vi "DeactivateChnl HW.vi"(8 "error in (no error)":errorcluster, 10 "Chnl Name":string, 11 "BME_DG_G08 in":refnum<class "BME_DG_G08.lvclass">) -> (0 "error out":errorcluster, 3 "BME_DG_G08 out":refnum<class "BME_DG_G08.lvclass">)   [LabVIEW 2009, in "POLARIS BME DG.lvlib" / "BME_DG_G08.lvclass"]
uses:
  BME_DG_G08.lvclass
  BME_DG_G05P2/BME_DG_G05P2.lvclass
  POLARIS BME DG.lvlib
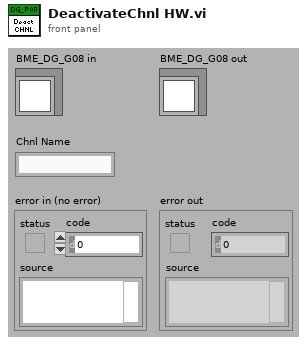
[diagram p1: front panel]
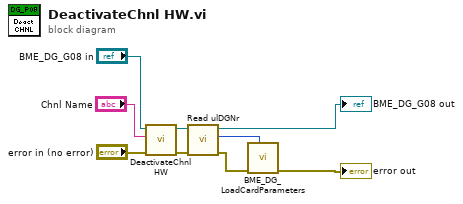
[diagram p0: block diagram]
diagram:
  n1 = call-parent "DeactivateChnl HW.vi"("error in (no error)"="error in (no error)", "Chnl Name"="Chnl Name", "BME_DG_Base in"="BME_DG_G08 in") -> ("error out"=w1:errorcluster, "BME_DG_Base out"=w2:refnum<class "BME_DG_G08.lvclass">)  [unwired: 7 in]
  n2 = call-dynamic "Read ulDGNr.vi"("error in (no error)"=w1, "BME_DG_Base in"=w2) -> ("error out"=w6:errorcluster, "ulDGNr"=w5:u32, "BME_DG_Base out"=→"BME_DG_G08 out":refnum<class "BME_DG_G08.lvclass">)  [unwired: 6 in, 1 out]
  n3 = call "BME_DG_LoadCardParameters.vi"("DG_Number"=w5, "error in (no error)"=w6) -> ("error out"=→"error out":errorcluster)  [unwired: 9 in]
